vi "RT Driver VI.vi"(7 "Operation":T1, 11 "Device Reference in":T2 format="%.0x") -> (0 "Error Code":i32)   [LabVIEW 2018, in "Instrument Addon Engine.lvlib"]
uses:
  Instrument Addon Engine.lvlib
  <vilib>/NI Veristand/Custom Device API/Custom Device Item Ref.ctl
  <vilib>/NI Veristand/Custom Device API/Hardware Interface Driver VI Operation.ctl
  <vilib>/NI/NIVS Inline Async API/_VS Inline Async API/VS Inline Async API/Types/Error Handling Settings.ctl
  Types/Commands RT Configuration Cluster.ctl
  Addon Shared/Types/Compiled Settings.ctl
  Addon Shared/Types/Command Parameters.ctl
  Addon Shared/Types/Linked Channel Cluster.ctl
  Addon Shared/Types/Command Channel Indeces.ctl
  Addon Shared/Types/Command Channel Index.ctl
  Addon Shared/Types/Response RT Configuration Cluster.ctl
  Addon Shared/Types/Response Parameters.ctl
  Addon Shared/Types/Response Wait Type.ctl
  Addon Shared/Types/Message Parameters.ctl
  Addon Shared/Types/Message Generation Type.ctl
  Addon Shared/Types/External Trigger Refs.ctl
  <vilib>/NI Veristand/Custom Device API/Data Reference.ctl
  Support Libraries/Protections.lvlibp/Parent Protection/Protection.lvclass
  Support Libraries/Protocols.lvlibp/Protocol Parent/Protocol Parent.lvclass
  <vilib>/NI/NIVS Inline Async API/_VS Inline Async API/VS Inline Async API/VS Inline Async API.lvclass
  <vilib>/NI/NIVS Inline Async API/_VS Inline Async API/VS Inline Async API/VS Inline Async API.lvclass/VS Inline Async API.ctl
  <vilib>/NI/NIVS Inline Async API/_Data Access Engine/Data Access Engine/Data Access Engine.lvclass/Data Access Engine.ctl
  <vilib>/NI/NIVS Inline Async API/_Data Access Engine/Access Type Classes/Write/Write.lvclass/Write.ctl
  <vilib>/NI/NIVS Inline Async API/_Data Access Engine/Access Type Classes/ReadWrite/ReadWrite.lvclass/ReadWrite.ctl
  <vilib>/NI/NIVS Inline Async API/_Data Access Engine/Access Type Classes/Read/Read.lvclass/Read.ctl
  <vilib>/NI/NIVS Inline Async API/_Data Access Engine/Data Access Engine/Methods/Data.Engine.Read Data from HW.vi
  <vilib>/NI/NIVS Inline Async API/_VS Inline Async API/Error Handling Process/SubVIs/Error.GetError.vi
  <vilib>/NI Veristand/Custom Device API/NI VeriStand - Get Channel Value by Data Reference.vi
  <vilib>/NI Veristand/Custom Device API/NI VeriStand - Set Channel Value by Data Reference.vi
  <vilib>/NI/NIVS Inline Async API/_Data Access Engine/Data Access Engine/Methods/Data.Engine.Write Data to HW.vi
  <vilib>/NI/NIVS Inline Async API/_Data Access Engine/Access Type Classes/ReadWrite/ReadWrite.EngineData.vi
  <vilib>/NI/NIVS Inline Async API/_Data Access Engine/Access Type Classes/Write/Write.EngineData.vi
  <vilib>/NI/NIVS Inline Async API/_Data Access Engine/Access Type Classes/Read/Read.EngineData.vi
  <vilib>/NI Veristand/Custom Device API/NI VeriStand - Get Channel Values by Block Data Reference.vi
  <vilib>/Utility/SystemLogging/Write to System Log.vi
  <vilib>/NI Veristand/Custom Device API/Global Data Refs.vi
  <vilib>/NI Veristand/Custom Device API/Custom Device API.lvlib
  Addon Shared/Instrument Addon Shared.lvlib
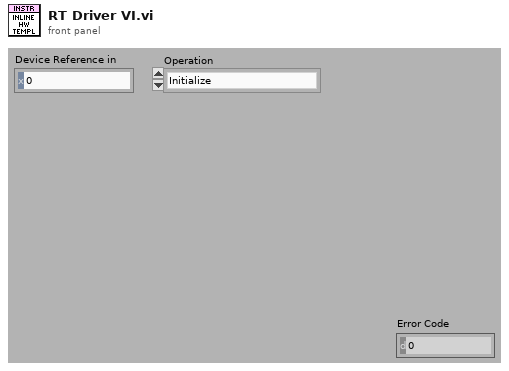
[diagram p1: front panel]
types:
  T1 = typedef "Custom Device API.lvlib/Hardware Interface Driver VI Operation.ctl" = enum16{"Initialize", "Start", "Read Data from HW", "Write Data to HW", "Close"}
  T2 = typedef "Custom Device API.lvlib/Custom Device Item Ref.ctl" = u64
  T3 = typedef "Instrument Addon Engine.lvlib/Commands RT Configuration Cluster.ctl" = cluster{"Compiled":T4, "Protection Settings":refnum<class "Protection.lvclass">[], "Protocol":refnum<class "Protocol Parent.lvclass">}
  T4 = typedef "Instrument Addon Shared.lvlib/Compiled Settings.ctl" = cluster{"Command Parameters":T5[], "Command Indeces":T7[], "MetaData Lookup":variant, "Name":string, "Data Lookup":variant, "Response Parameters":T9[], "Message Generation Settings":T12[], "Wait Value Lookup":variant, "Decimation":u32, "External Channels":T14}
  T5 = typedef "Instrument Addon Shared.lvlib/Command Parameters.ctl" = cluster{"Command":string, "Linked Channels":T6[], "Pad":bool, "Length":u32, "Pad Value":u8}
  T6 = typedef "Instrument Addon Shared.lvlib/Linked Channel Cluster.ctl" = cluster{"Variable Name":string, "GUID":string}
  T7 = typedef "Instrument Addon Shared.lvlib/Command Channel Indeces.ctl" = cluster{"Channels":T8[]}
  T8 = typedef "Instrument Addon Shared.lvlib/Command Channel Index.ctl" = cluster{"Data Index":i32, "Data Length":i32}
  T9 = typedef "Instrument Addon Shared.lvlib/Response RT Configuration Cluster.ctl" = cluster{"Reponse Parameters":T10, "Use?":bool}
  T10 = typedef "Instrument Addon Shared.lvlib/Response Parameters.ctl" = cluster{"Response":string, "Linked Channels":T6[], "Type Value":dbl, "Wait Type":T11, "Use Channel":bool, "Channel Path":string}
  T11 = typedef "Instrument Addon Shared.lvlib/Response Wait Type.ctl" = enum16{"Byte Count", "Wait sec"}
  T12 = typedef "Instrument Addon Shared.lvlib/Message Parameters.ctl" = cluster{"Generation Type":T13, "Period":dbl, "Include Protection":bool, "Type":string}
  T13 = typedef "Instrument Addon Shared.lvlib/Message Generation Type.ctl" = enum16{"Trigger Only", "Periodic & Trigger", "Value Change & Trigger"}
  T14 = typedef "Instrument Addon Shared.lvlib/External Trigger Refs.ctl" = cluster{"Channels":T15[], "Triggers":T15[], "Values":dbl[]}
  T15 = typedef "Custom Device API.lvlib/Data Reference.ctl" = i32
  T16 = cluster{"Settings":T3, "Processes":refnum<class "VS Inline Async API.lvclass">}
  T17 = typedef "VS Inline Async API.lvlib/VS Inline Async API.lvclass/Error Handling Settings.ctl" = cluster{"Write to SystemLog (F)":bool}
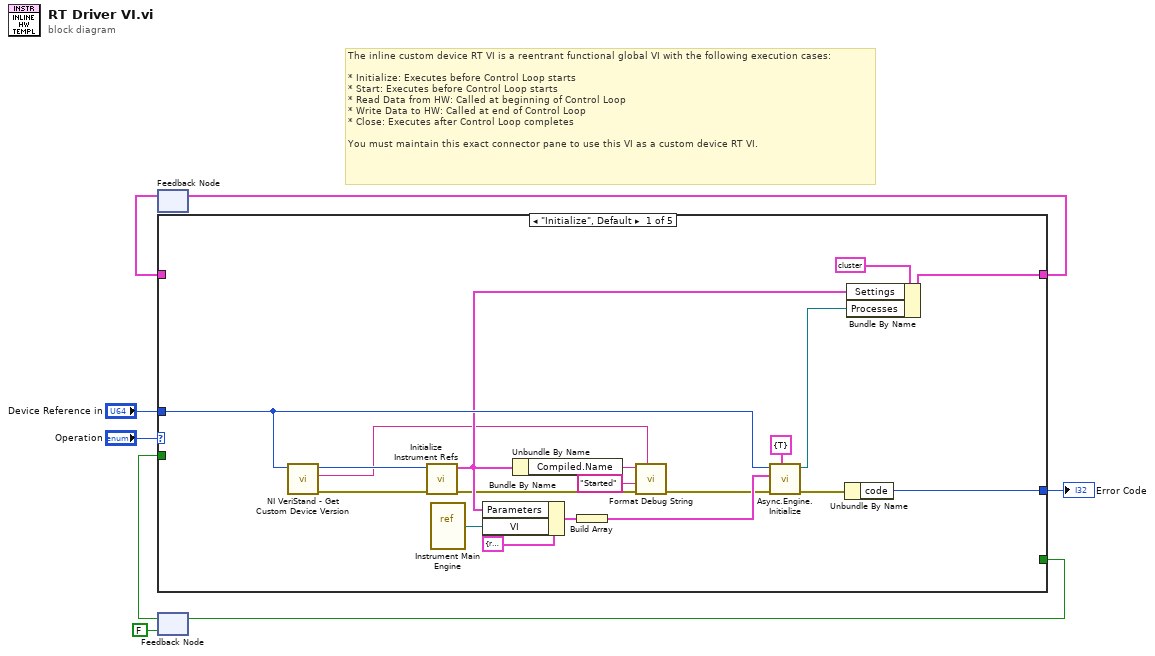
[diagram p0: block diagram]
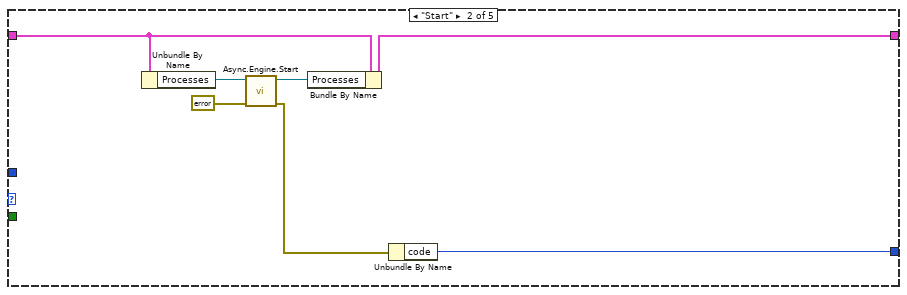
[diagram p2: hidden frame]
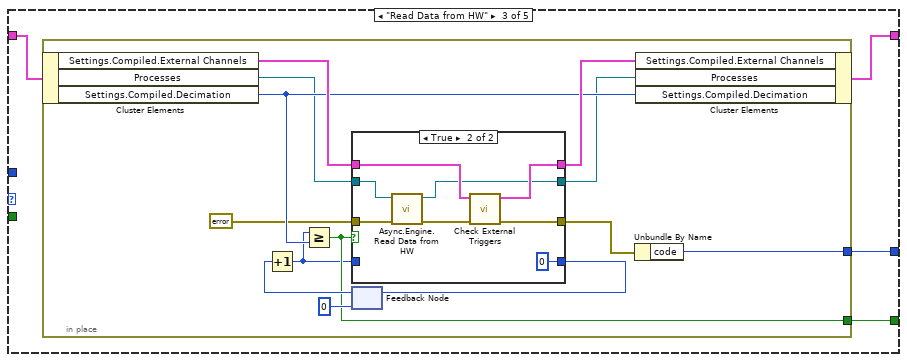
[diagram p3: hidden frame]
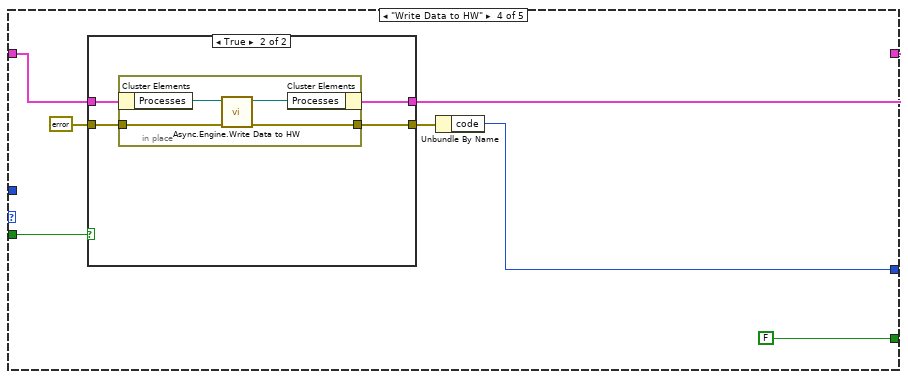
[diagram p5: hidden frame]
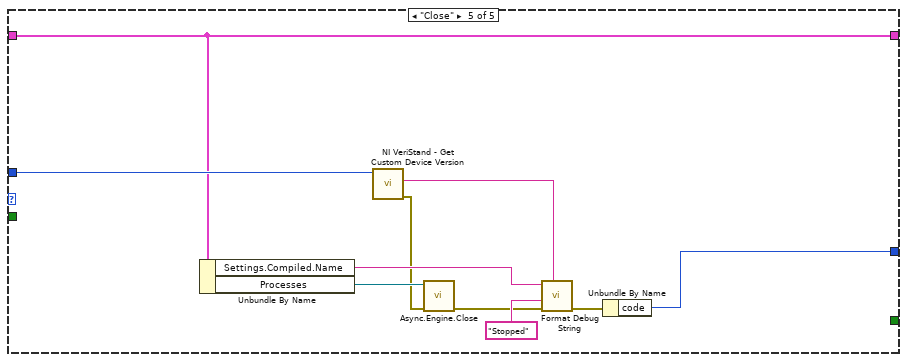
[diagram p7: hidden frame]
diagram:
  # "The inline custom device RT VI is a reentrant functional global VI with the following execution cases:\n\n* Initialize: Executes before Control Loop starts\n* Start: Executes before Control Loop starts\n* Read Data from HW: Called at beginning of Control Loop\n* Write Data to HW: Called at end of Control Loop\n* Close: Executes after Control Loop completes\n\nYou must maintain this exact connector pane to use this VI as a custom device RT VI."
  n1 = feedback #1() -> (w6:T16)  [unwired: 1 out]
  n2 = feedback #2(FALSE) -> (w2:bool)
  n3 = case shown="\"Initialize\", Default" "Operation" {
    tunnel: [w26 w32 w36 w70 w84] -> w7
    tunnel: w6 -> [_ w33 w37 w69 w84]
    tunnel: "Device Reference in" -> [w19 _ _ _ w87]
    tunnel: [w27 w34 w35 w65 w82] -> w4
    tunnel: [_ _ w38 FALSE _] -> w3
    tunnel: w2 -> [_ _ _ w68 _]
    frame "Initialize", Default {
      n4 = call <vilib>:"NI VeriStand - Get Custom Device Version.vi"("Device Ref in"=w19) -> ("error out"=w17:errorcluster, "Value"=w14:string, "Device Ref out"=w18:T2)  [unwired: 8 in]
      n5 = call "Initialize Instrument Refs.vi"("error in (no error)"=w17, "Device Reference in"=w18) -> ("error out"=w11:errorcluster, "Settings"=w16:T3)  [unwired: 8 in]
      n6 = vi-ref "Instrument Main Engine.vi"() -> (w23:refnum<vi>)
      n7 = Bundle By Name(cluster=cluster{"VI":refnum<vi>, "Parameters":variant} {"VI"=refnum, "Parameters"=variant} ("Process"), "Parameters"=w16, "VI"=w23) -> (w22:cluster{"VI":refnum<vi>, "Parameters":variant})
      n8 = Unbundle By Name(w16) -> ("Compiled.Name"=w13:string)
      n9 = Build Array(w22) -> (w21:cluster{"VI":refnum<vi>, "Parameters":variant}[])
      n10 = call "Format Debug String.vi"("Version"=w14, "error in (no error)"=w11, "State"="Started" ("string"), "Name"=w13) -> ("error out"=w10:errorcluster)  [unwired: 6 in, 1 out]
      n11 = call <vilib>:"Async.Engine.Initialize.vi"("Error Log Settings"=T17 {"Write to SystemLog (F)"=TRUE}, "error in (no error)"=w10, "Processes"=w21, "Custom Device Ref"=w19) -> ("error out"=w25:errorcluster, "Async"=w20:refnum<class "VS Inline Async API.lvclass">)  [unwired: 6 in]
      n12 = Unbundle By Name(w25) -> ("code"=w27:i32)
      n13 = Bundle By Name(cluster=T16 {"Settings"={"Compiled"={"Command Parameters"=[], "Command Indeces"=[], "MetaData Lookup"=variant, "Name"="", "Data Lookup"=variant, "Response Parameters"=[], "Message Generation Settings"=[], "Wait Value Lookup"=variant, "Decimation"=0, "External Channels"={"Channels"=[], "Triggers"=[], "Values"=[]}}, "Protection Settings"=[], "Protocol"=refnum}, "Processes"=refnum}, "Settings"=w16, "Processes"=w20) -> (w26:T16)
    }
    frame "Start" {
      n14 = Unbundle By Name(w33) -> ("Processes"=w31:refnum<class "VS Inline Async API.lvclass">)
      n15 = call <vilib>:"Async.Engine.Start.vi"("error in (no error)"=errorcluster {"status"=FALSE, "code"=0, "source"=""} ("error in"), "VS Inline Async API in"=w31) -> ("error out"=w29:errorcluster, "VS Inline Async API out"=w30:refnum<class "VS Inline Async API.lvclass">)  [unwired: 8 in]
      n16 = Bundle By Name(cluster=w33, "Processes"=w30) -> (w32:T16)
      n17 = Unbundle By Name(w29) -> ("code"=w34:i32)
    }
    frame "Read Data from HW" {
      n18 = in-place {
        in-place-border: [w49] -> w38
        in-place-border: [w40] -> w35
        n19 = in-place-cluster #3(w37) -> ("Settings.Compiled.External Channels"=w48:T14, "Processes"=w44:refnum<class "VS Inline Async API.lvclass">, "Settings.Compiled.Decimation"=w46:u32)
        n20 = feedback #4(u32 0) -> (w50:u32)
        n21 = Increment(x=w50) -> (x+1=w42:u32)
        n22 = Greater Or Equal?(x=w42, y=w46) -> (x >= y?=w49:bool)
        n23 = case shown="True" w49 {
          tunnel: [w52 w63] -> w41
          tunnel: w48 -> [w55 w62]
          tunnel: [w55 w61] -> w47
          tunnel: [w54 w59] -> w45
          tunnel: w44 -> [w54 w58]
          tunnel: [w53 u32 0] -> w43
          tunnel: w42 -> [w53 _]
          tunnel: errorcluster {"status"=FALSE, "code"=0, "source"=""} ("error in") -> [w52 w56]
          frame False {
          }
          frame True {
            n24 = call <vilib>:"Async.Engine.Read Data from HW.vi"("error in"=w56, "Async in"=w58) -> ("error out"=w60:errorcluster, "Async out"=w59:refnum<class "VS Inline Async API.lvclass">)  [unwired: 8 in]
            n25 = call "Check External Triggers.vi"("error in (no error)"=w60, "Refs"=w62) -> ("error out"=w63:errorcluster, "Refs"=w61:T14)  [unwired: 8 in]
          }
        }
        n26 = feedback-in #4(w43) -> ()
        n27 = Unbundle By Name(w41) -> ("code"=w40:i32)
        n28 = in-place-cluster #3("Settings.Compiled.External Channels"=w47, "Processes"=w45, "Settings.Compiled.Decimation"=w46) -> (w36:T16)
      }
    }
    frame "Write Data to HW" {
      n29 = case shown="True" w68 {
        tunnel: [w72 w75] -> w70
        tunnel: w69 -> [w72 w76]
        tunnel: [w71 w74] -> w66
        tunnel: errorcluster {"status"=FALSE, "code"=0, "source"=""} ("error in") -> [w71 w73]
        frame False {
        }
        frame True {
          n30 = in-place {
            in-place-border: [w78] -> w74
            in-place-border: w73 -> [w77]
            n31 = in-place-cluster #5(w76) -> ("Processes"=w80:refnum<class "VS Inline Async API.lvclass">)
            n32 = call <vilib>:"Async.Engine.Write Data to HW.vi"("error in (no error)"=w77, "VS Inline Async API in"=w80) -> ("error out"=w78:errorcluster, "VS Inline Async API out"=w79:refnum<class "VS Inline Async API.lvclass">)  [unwired: 8 in]
            n33 = in-place-cluster #5("Processes"=w79) -> (w75:T16)
          }
        }
      }
      n34 = Unbundle By Name(w66) -> ("code"=w65:i32)
    }
    frame "Close" {
      n35 = Unbundle By Name(w84) -> ("Settings.Compiled.Name"=w86:string, "Processes"=w90:refnum<class "VS Inline Async API.lvclass">)
      n36 = call <vilib>:"NI VeriStand - Get Custom Device Version.vi"("Device Ref in"=w87) -> ("error out"=w81:errorcluster, "Value"=w89:string)  [unwired: 8 in, 1 out]
      n37 = call <vilib>:"Async.Engine.Close.vi"("error in (no error)"=w81, "Async in"=w90) -> ("error out"=w85:errorcluster)  [unwired: 8 in, 1 out]
      n38 = call "Format Debug String.vi"("Version"=w89, "error in (no error)"=w85, "State"="Stopped" ("string"), "Name"=w86) -> ("error out"=w83:errorcluster)  [unwired: 6 in, 1 out]
      n39 = Unbundle By Name(w83) -> ("code"=w82:i32)
    }
  }
  "Error Code" <- w4
  n40 = feedback-in #1(w7) -> ()
  n41 = feedback-in #2(w3) -> ()
